vi "Spatial Dual Decode Packet 85 (SubVI).vi"(8 "SGL Precision":i16=6, 10 "Packet 85 Bytes In":u8[](array[numeric])) -> (0 "Channel Data Type":string[](array[string])=["Float", "Float", "Float"], 1 "Channel Units":string[](array[string])=["m/s/s", "m/s/s", "m/s/s"], 2 "Data":string[](array[string]), 3 "Channel Names":string[](array[string])=["Acc X", "Acc Y", "Acc Z"], 4 "Packet 85 Decoded Data Cluster":T1)   [LabVIEW 2019, in "SpatialDual_Parsers.lvlib"]
uses:
  SpatialDual_Parsers.lvlib
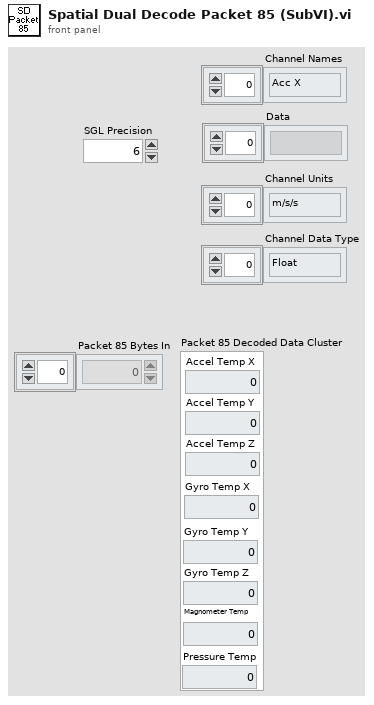
[diagram p1: front panel]
types:
  T1 = cluster{"Accel Temp X":sgl, "Accel Temp Y":sgl, "Accel Temp Z":sgl, "Gyro Temp X":sgl, "Magnometer Temp":sgl, "Gyro Temp Z":sgl, "Gyro Temp Y":sgl, "Pressure Temp":sgl}
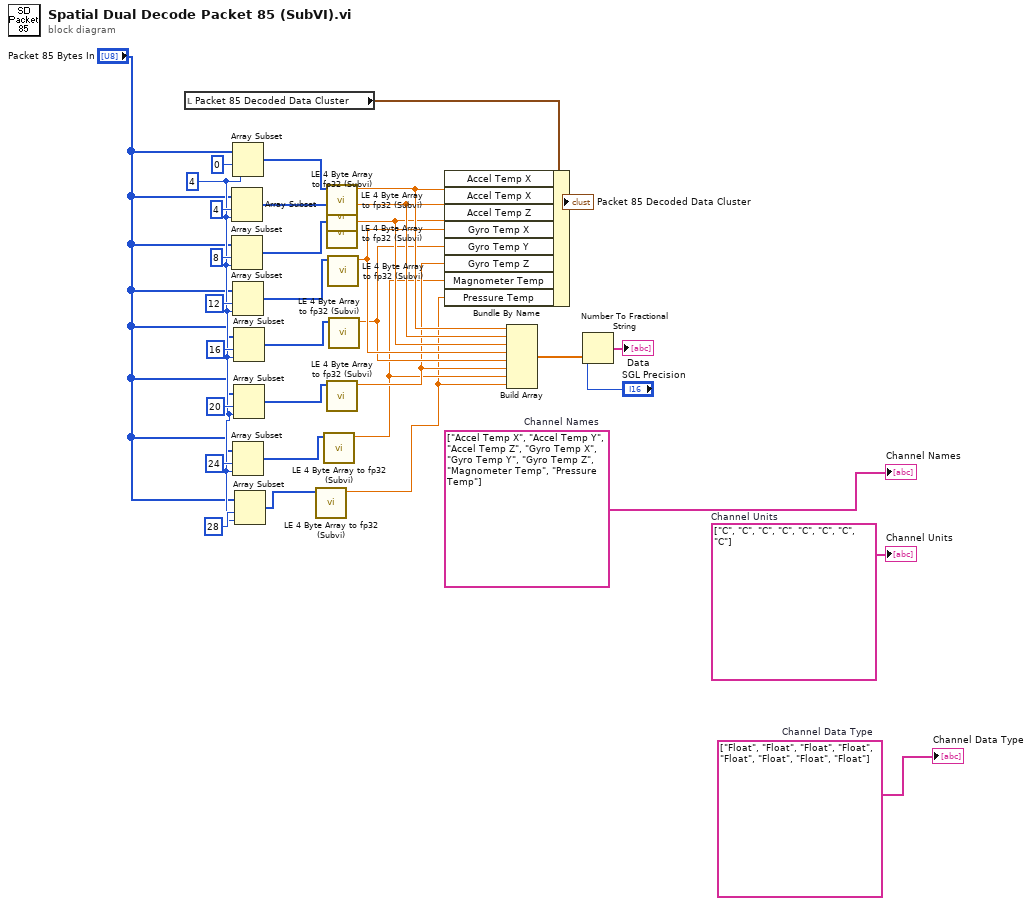
[diagram p0: block diagram]
diagram:
  w19 = string[] ["Float", "Float", "Float", "Float", "Float", "Float", "Float", "Float"]  # Channel Data Type
  w20 = string[] ["C", "C", "C", "C", "C", "C", "C", "C"]  # Channel Units
  w21 = string[] ["Accel Temp X", "Accel Temp Y", "Accel Temp Z", "Gyro Temp X", "Gyro Temp Y", "Gyro Temp Z", "Magnometer Temp", "Pressure Temp"]  # Channel Names
  w11 = 4 ("length")
  n1 = local read "Packet 85 Decoded Data Cluster"() -> (w34:T1)
  n2 = Array Subset(array="Packet 85 Bytes In", index=4, length=w11) -> (w28:u8[])
  n3 = Array Subset(array="Packet 85 Bytes In", index=8, length=w11) -> (w29:u8[])
  n4 = Array Subset(array="Packet 85 Bytes In", index=0, length=w11) -> (w27:u8[])
  n5 = Array Subset(array="Packet 85 Bytes In", index=12, length=w11) -> (w17:u8[])
  n6 = Array Subset(array="Packet 85 Bytes In", index=24, length=w11) -> (w7:u8[])
  n7 = Array Subset(array="Packet 85 Bytes In", index=16, length=w11) -> (w9:u8[])
  n8 = Array Subset(array="Packet 85 Bytes In", index=20, length=w11) -> (w8:u8[])
  n9 = Array Subset(array="Packet 85 Bytes In", index=28, length=w11) -> (w6:u8[])
  n10 = call "LE 4 Byte Array to fp32 (Subvi).vi"("4 Bytes in"=w6) -> ("fp32 Out"=w1:sgl)  [unwired: 8 in]
  n11 = call "LE 4 Byte Array to fp32 (Subvi).vi"("4 Bytes in"=w7) -> ("fp32 Out"=w2:sgl)  [unwired: 8 in]
  n12 = call "LE 4 Byte Array to fp32 (Subvi).vi"("4 Bytes in"=w27) -> ("fp32 Out"=w26:sgl)  [unwired: 8 in]
  n13 = call "LE 4 Byte Array to fp32 (Subvi).vi"("4 Bytes in"=w28) -> ("fp32 Out"=w25:sgl)  [unwired: 8 in]
  n14 = call "LE 4 Byte Array to fp32 (Subvi).vi"("4 Bytes in"=w29) -> ("fp32 Out"=w24:sgl)  [unwired: 8 in]
  n15 = call "LE 4 Byte Array to fp32 (Subvi).vi"("4 Bytes in"=w8) -> ("fp32 Out"=w3:sgl)  [unwired: 8 in]
  n16 = call "LE 4 Byte Array to fp32 (Subvi).vi"("4 Bytes in"=w17) -> ("fp32 Out"=w16:sgl)  [unwired: 8 in]
  n17 = call "LE 4 Byte Array to fp32 (Subvi).vi"("4 Bytes in"=w9) -> ("fp32 Out"=w4:sgl)  [unwired: 8 in]
  n18 = Bundle By Name(cluster=w34, "Accel Temp X"=w26, "Accel Temp X"=w25, "Accel Temp Z"=w24, "Gyro Temp X"=w16, "Gyro Temp Y"=w4, "Gyro Temp Z"=w3, "Magnometer Temp"=w2, "Pressure Temp"=w1) -> (→"Packet 85 Decoded Data Cluster":T1)
  n19 = Build Array(w26, w25, w24, w16, w4, w3, w2, w1) -> (w5:sgl[])
  n20 = Number To Fractional String(number=w5, precision (6)="SGL Precision") -> (F-format string=→"Data":string[])  [unwired: 2 in]
  "Channel Names" <- w21
  "Channel Units" <- w20
  "Channel Data Type" <- w19
